vi "NOAH.vi"() -> ()   [LabVIEW 2017]
panel:
  out "WT-40":dbl
  out "BT-41":dbl
  out "BT-30":dbl
  out "WT-31":dbl
  out "Calculation vs. Reading 2":dbl(graph)
  in  "Fault Text 2":string
  out "Pump Light 2":bool
  out "Frequency [Hz] 2":u16(knob) scale=0.0..230.0
  out "Posting Time 2":timestamp format="%<%H:%M:%S>T"
  out "Time to Handle 2":timestamp format="%<%H:%M:%S>T"
  out "Fault Priority Rank 2":dbl
  out "Calculation vs. Reading":dbl(graph)
  in  "Fault Text":string
  out "Pump Light":bool
  out "Frequency [Hz]":u16(knob) scale=0.0..230.0
  out "Posting Time":timestamp format="%<%H:%M:%S>T"
  out "Time to Handle":timestamp format="%<%H:%M:%S>T"
  out "Fault Priority Rank":dbl
  out "Notification Light":bool
  out "OK Time":timestamp format="%<%H:%M:%S>T"
  in  "Problem Count":dbl
  in  "Prompt Count":dbl
  in  "Warning Count":dbl
  in  "Total Notifications":dbl format="%#.0g"
  # "At-a-Glance"
  # "Fault Information"
  # "Priority"
  # "to handle"
  # "PUMP"
  # "Posted at"
  # "Pinned Items"
  # "Analytics"
  # "Priority"
  # "to handle"
  # "PUMP"
  # "Posted at"
  # "Model HQ"
  # "Analytical"
  # "Grey-Box"
  # "Data-Driven"
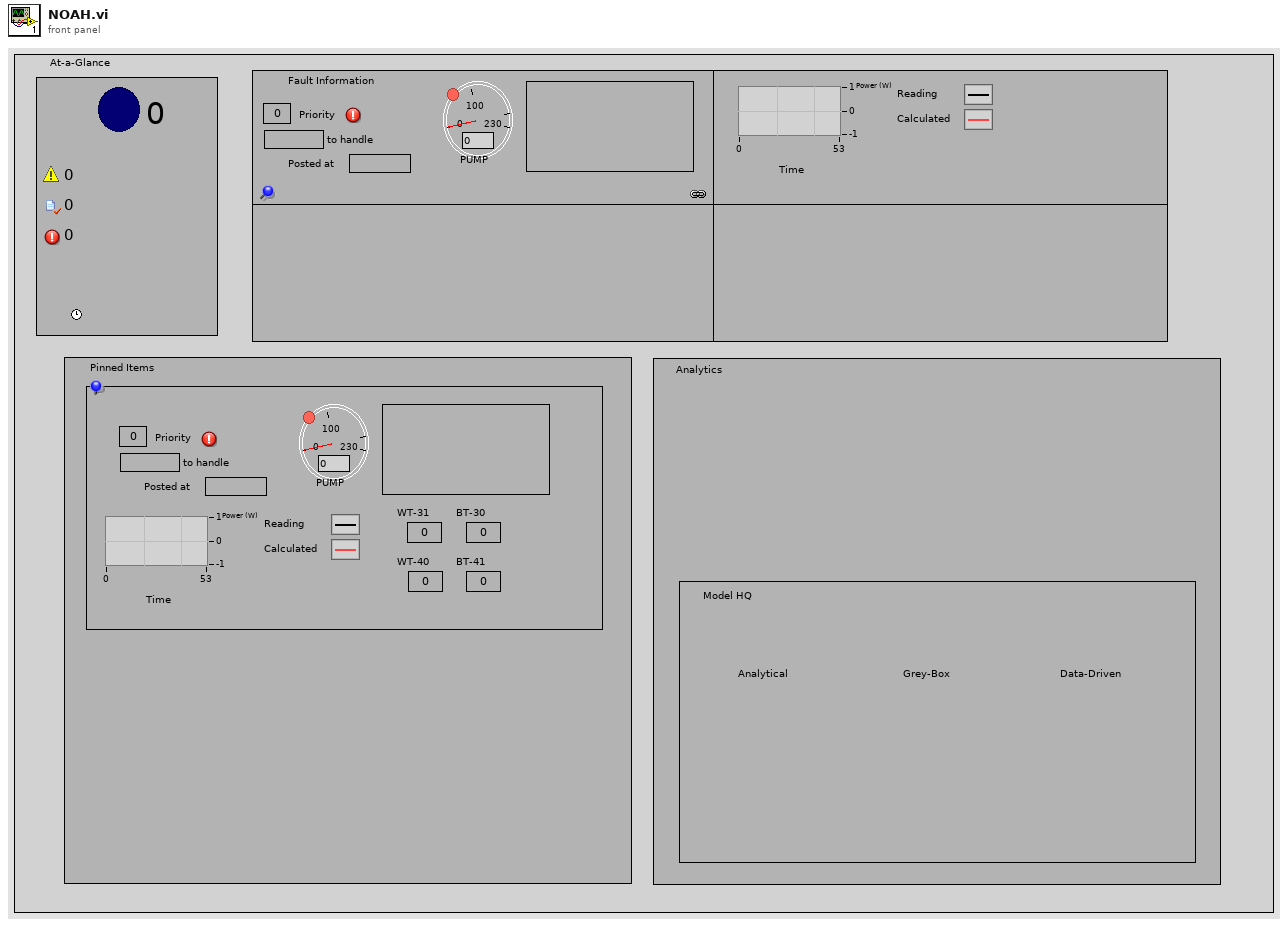
[diagram p1: front panel]
types:
  T1 = cluster{"timestamps":timestamp[], "data":dbl[]}[]
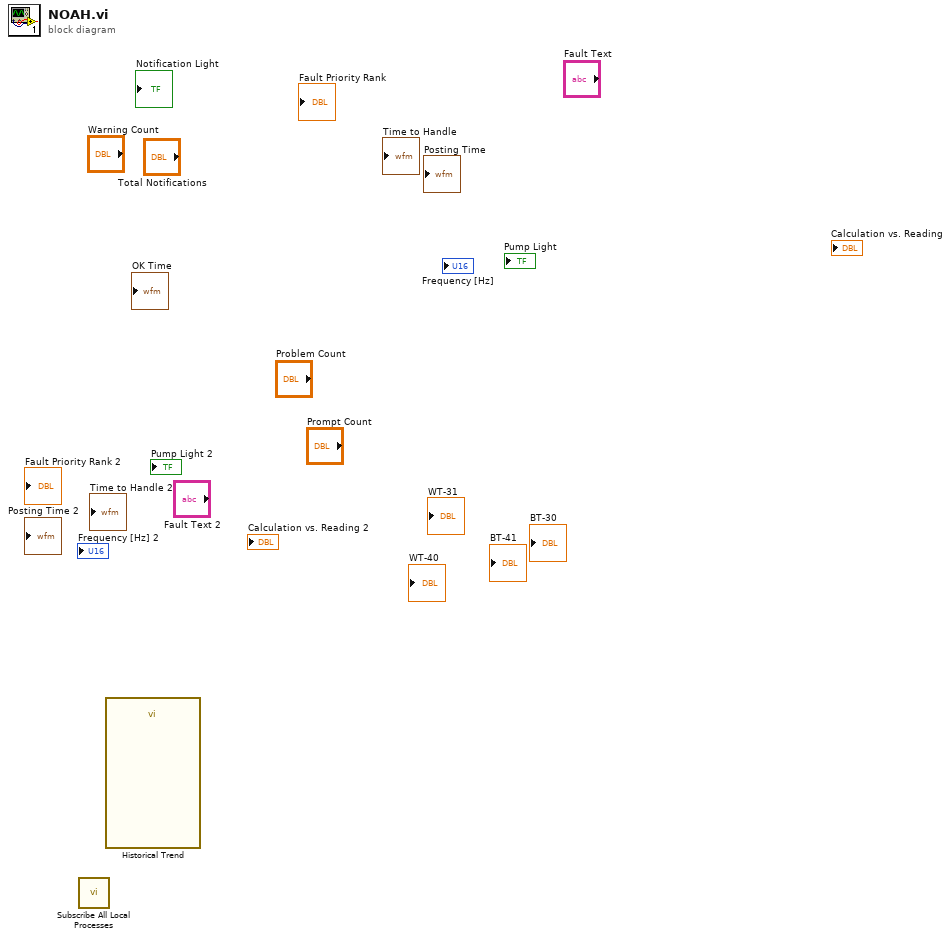
[diagram p0: block diagram]
diagram:
  n1 = call <vilib>:"Subscribe All Local Processes.vi"() -> ("Alarm & Event Displayer reference"=w1:refnum<k7>)  [unwired: 9 in, 2 out]
  n2 = call "Historical Trend"() -> ("Historical Traces"=w3:T1, "Trend Reference"=w2:refnum<vi>)  [unwired: 7 in, 3 out]
